vi "Controls Loop.vi"(8 "error in":errorcluster, 10 "Controls[]":refnum<vi>[](array[refnum]), 11 "Material-Scheme in":refnum<class "Material-Scheme.lvclass">) -> (0 "error out":errorcluster)   [LabVIEW 2021, in "TSC Material Theme.lvlib" / "Material-Scheme.lvclass"]
doc: "loop through all the controls on a panel in order to change the appearance\n\n<b>Code Developed By:</b> +\nDaniel Coons +\nTechnology Service Corporation +\nwww.tsc.com/atcs"
uses:
  Material-Scheme.lvclass
  Material-Scheme.lvclass/Material-Scheme.ctl
  <vilib>/Utility/miscctls.llb/LVRowAndColumnTypeDef.ctl
  data member access/Get name.vi
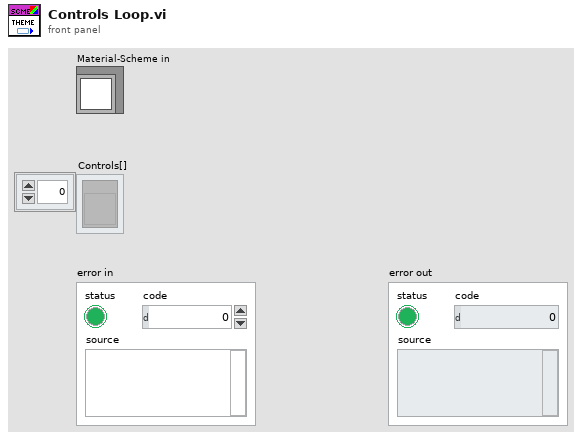
[diagram p1: front panel]
types:
  T1 = typedef "LVRowAndColumnTypeDef.ctl" = cluster{"Row":i32, "Column":i32}
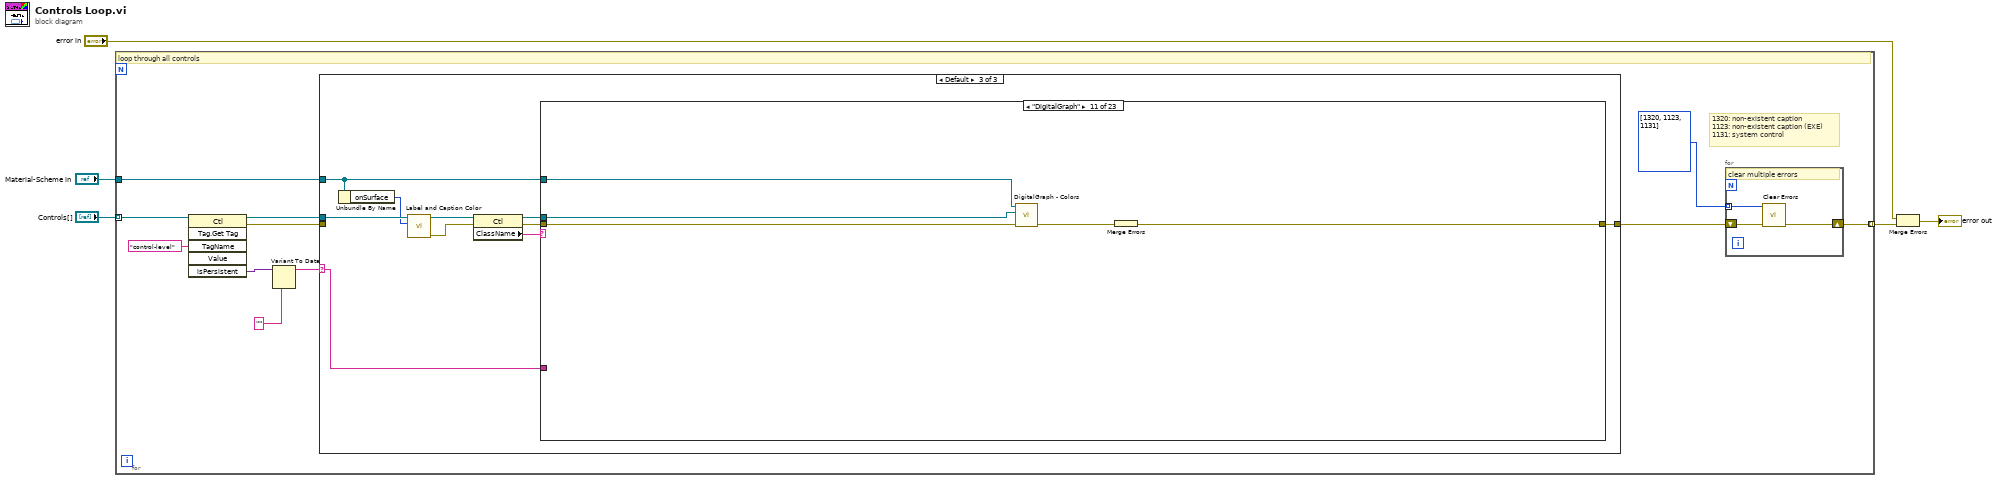
[diagram p0: block diagram]
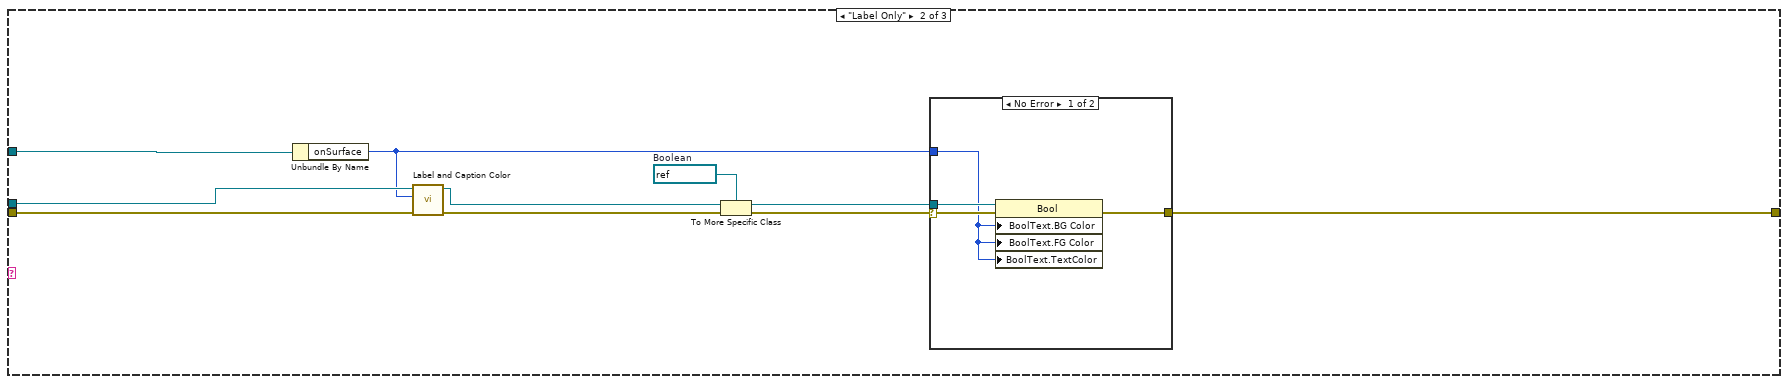
[diagram p3: hidden frame]
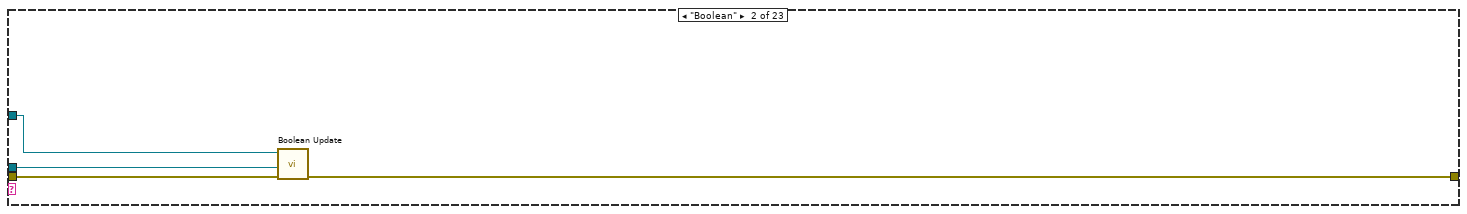
[diagram p6: hidden frame]
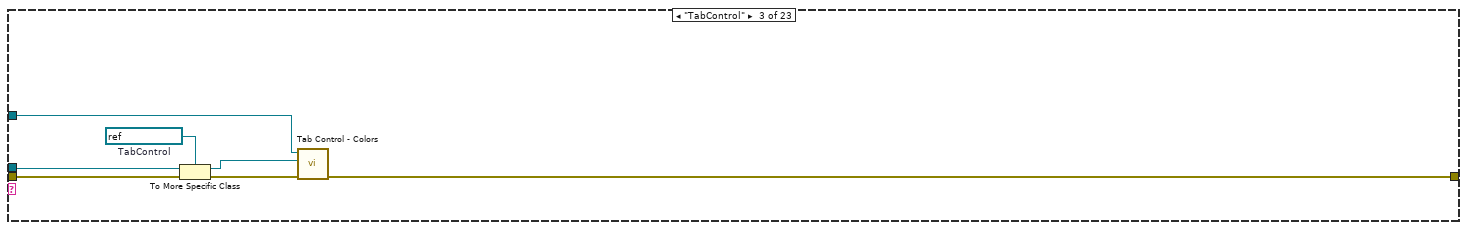
[diagram p7: hidden frame]
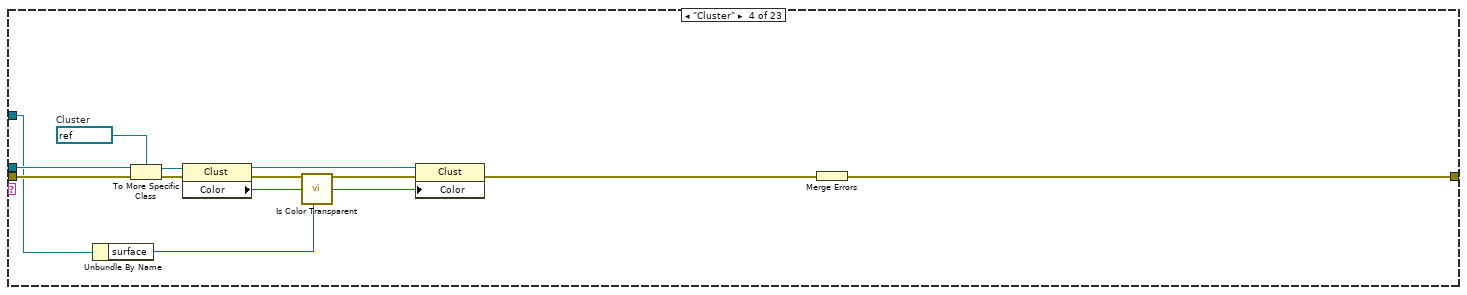
[diagram p8: hidden frame]
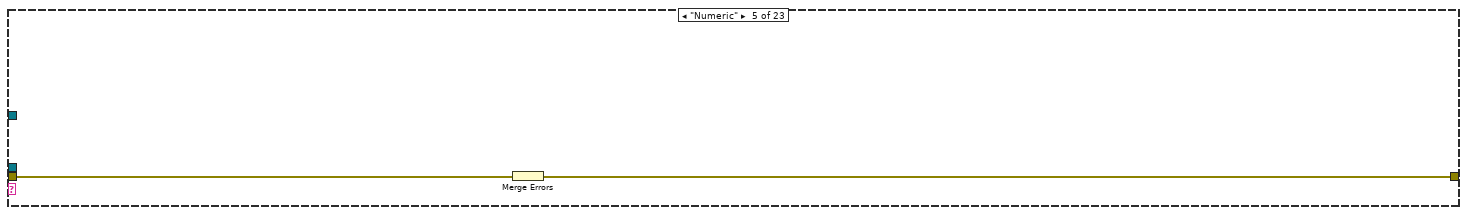
[diagram p9: hidden frame]
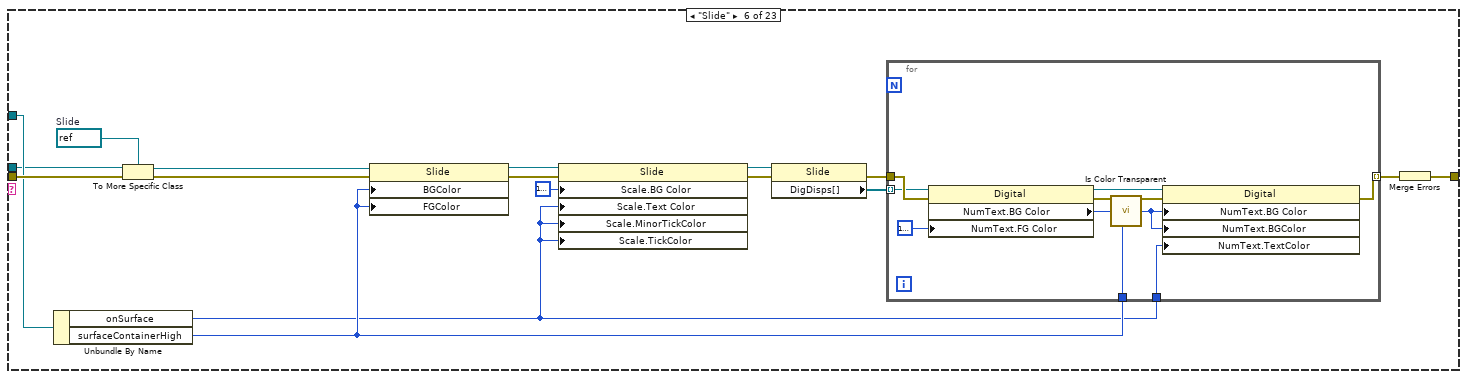
[diagram p10: hidden frame]
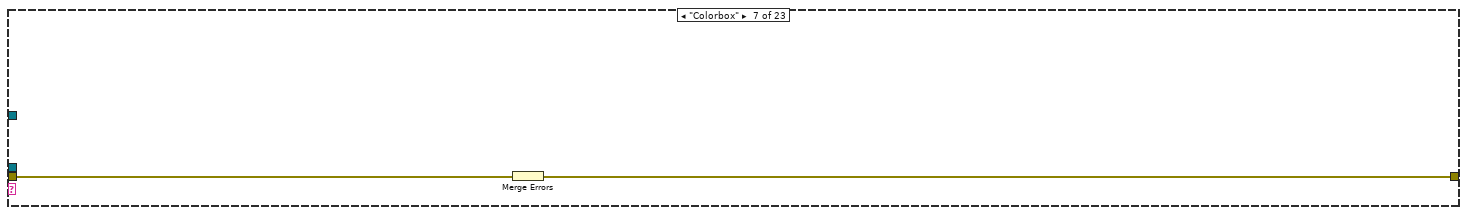
[diagram p11: hidden frame]
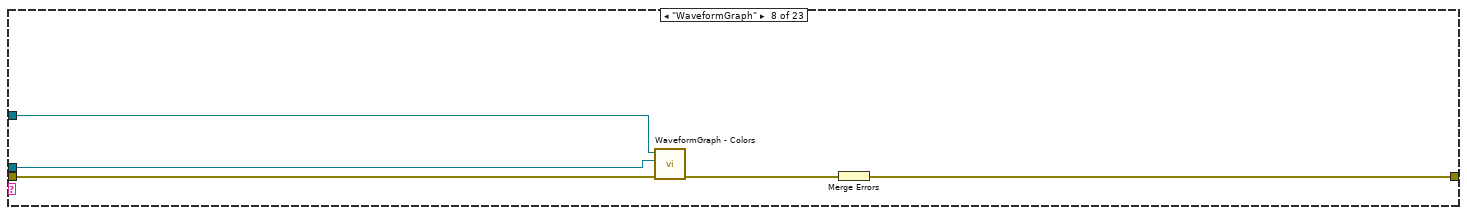
[diagram p12: hidden frame]
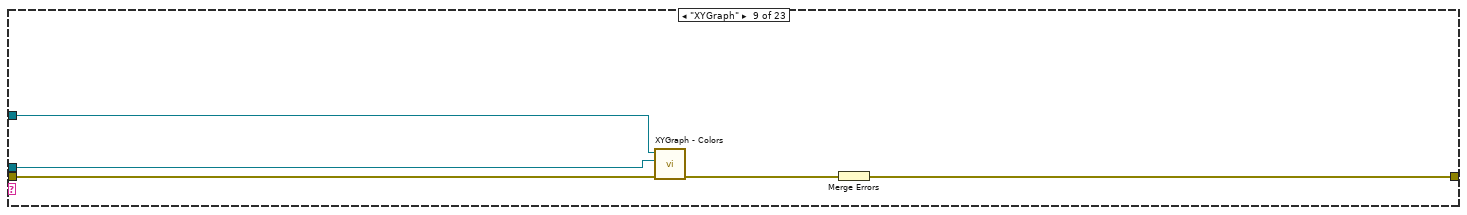
[diagram p13: hidden frame]
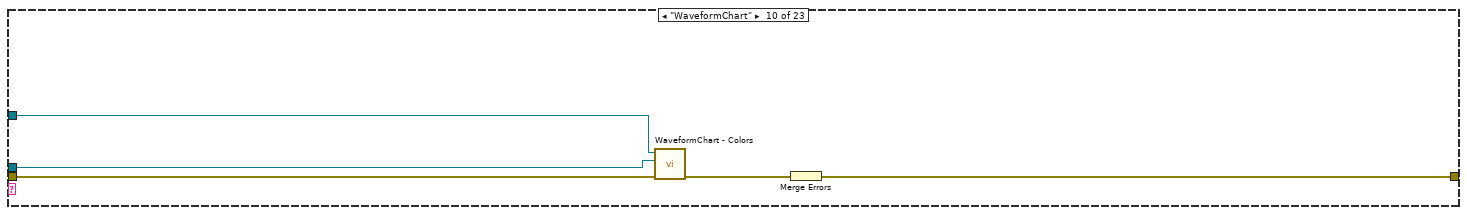
[diagram p14: hidden frame]
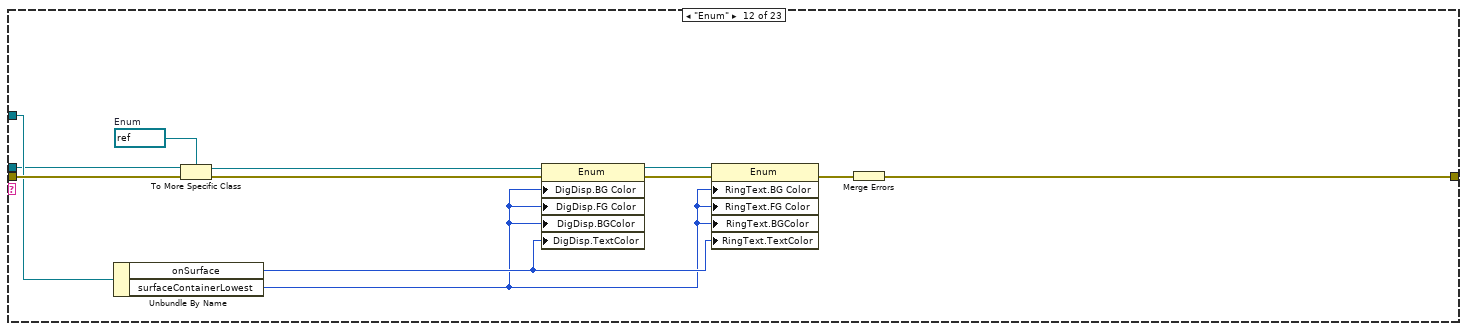
[diagram p15: hidden frame]
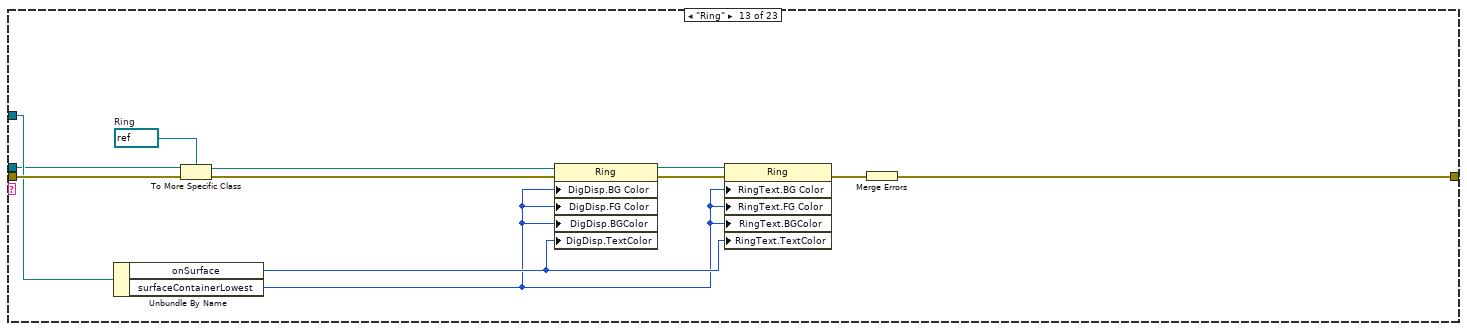
[diagram p16: hidden frame]
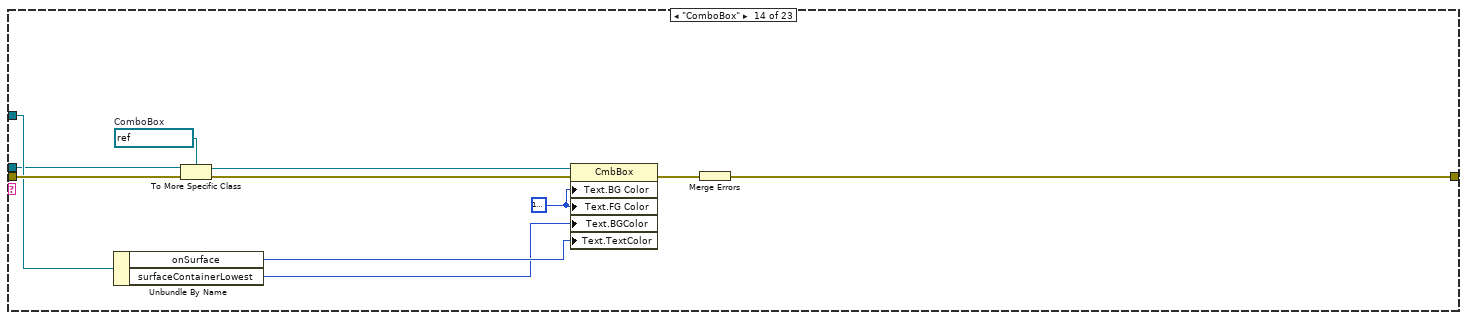
[diagram p17: hidden frame]
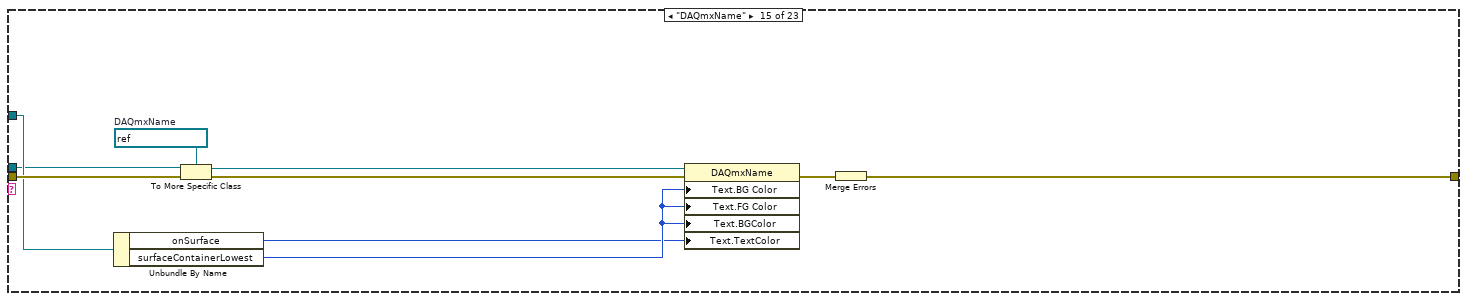
[diagram p18: hidden frame]
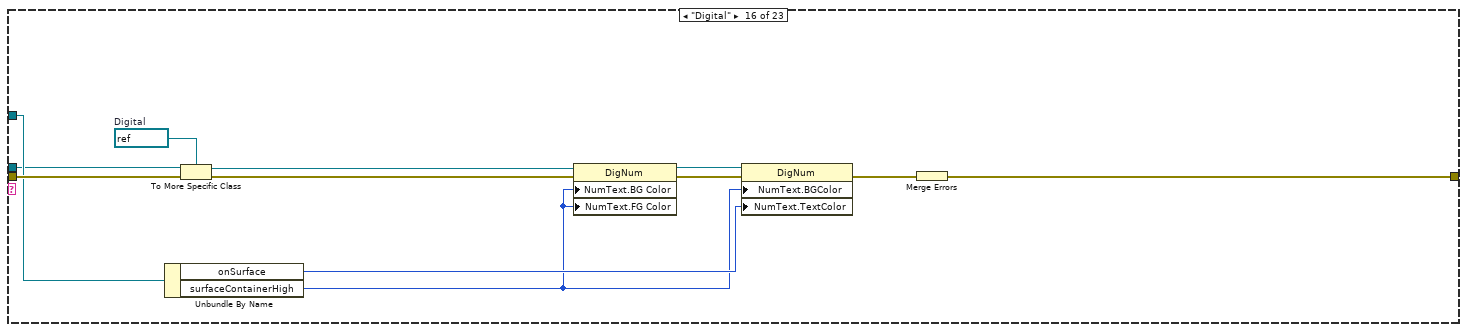
[diagram p19: hidden frame]
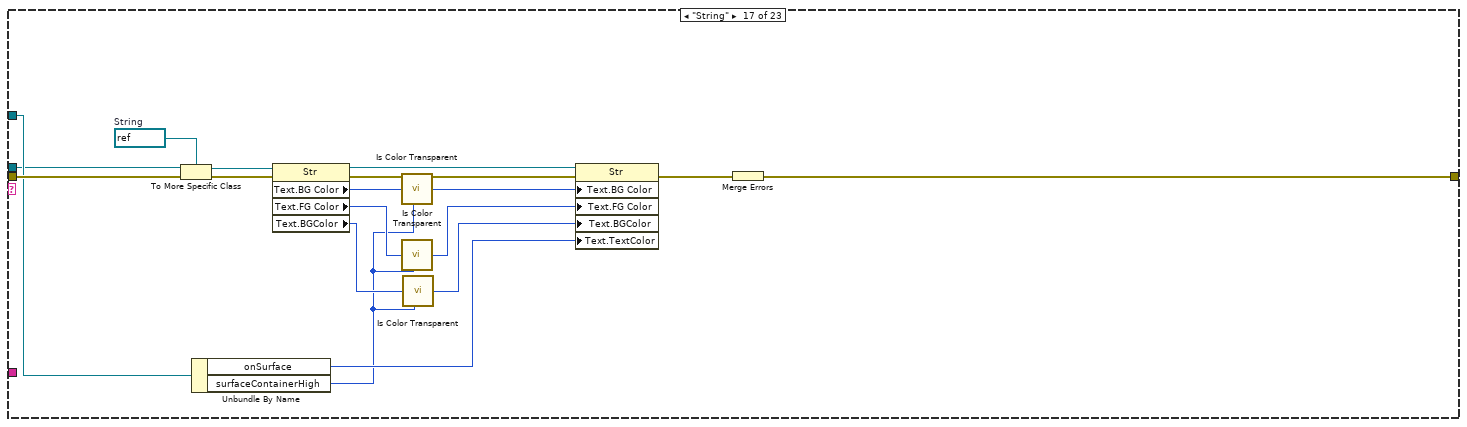
[diagram p20: hidden frame]
diagram:
  n1 = for {
    tunnel: "Controls[]" -> [w13] mode=indexing
    tunnel: "Material-Scheme in" -> [w16]
    tunnel: [w7] -> w3 mode=indexing
    # "1320: non-existent caption\n1123: non-existent caption (EXE)\n1131: system control"
    # "loop through all controls"
    n2 = invoke class="Ctl" method="Tag.Get Tag"(reference=w13, "TagName"="control-level" ("Tag Name")) -> (reference out=w12:refnum<vi>, error out=w8:errorcluster, "isPersistent"=w11:variant)  [unwired: 4 in, 3 out]
    n3 = Variant To Data(type="", Variant=w11) -> (data=w9:string)  [unwired: 1 in, 1 out]
    n4 = case shown="Default" w9 {
      selector: w9 -> [_ _ w37]
      tunnel: w12 -> [_ w20 w36]
      tunnel: w16 -> [_ w26 w33]
      tunnel: [w17 w22 w38] -> w15
      tunnel: w8 -> [w17 w27 _]
      frame "N/A", "no change", "no-change" {
      }
      frame "Label Only" {
        w25 = refnum<vi> refnum  # Boolean
        n5 = Unbundle By Name(w26) -> ("onSurface"=w18:u32)
        n6 = call "Label and Caption Color.vi"("error in"=w27, "Text Color"=w18, "ctrl ref in"=w20) -> ("error out"=w21:errorcluster, "ctrl ref out"=w19:refnum<vi>)  [unwired: 7 in]
        n7 = To More Specific Class(target class=w25, reference=w19, error in=w21) -> (specific class reference=w24:refnum<vi>, error out=w23:errorcluster)
        n8 = case shown="No Error" w23 {
          selector: w23 -> [w30 _]
          tunnel: w24 -> [w31 _]
          tunnel: w18 -> [w29 _]
          tunnel: [w28 _] -> w22
          frame No Error {
            n9 = property class="Bool"(reference=w31, error in=w30, "BoolText.BG Color"=w29, "BoolText.FG Color"=w29, "BoolText.TextColor"=w29) -> (error out=w28:errorcluster)  [unwired: 1 out]
          }
          frame Error {
          }
        }
      }
      frame Default {
        n10 = Unbundle By Name(w33) -> ("onSurface"=w32:u32)
        n11 = call "Label and Caption Color.vi"("Text Color"=w32, "ctrl ref in"=w36) -> ("error out"=w34:errorcluster, "ctrl ref out"=w35:refnum<vi>)  [unwired: 8 in]
        n12 = property class="Ctl"(reference=w35, error in=w34) -> (reference out=w40:refnum<vi>, error out=w39:errorcluster, "ClassName"=w41:string)
        n13 = case shown="\"DigitalGraph\"" w41 {
          tunnel: w40 -> [_ w43 w49 w65 _ w83 _ w99 w104 w109 w114 w125 w137 w148 w158 w170 w187 w196 w206 w217 w239 w266 w286]
          tunnel: w39 -> [w42 w46 w50 w64 w68 w85 w97 w102 w107 w112 w117 w129 w141 w152 w162 w174 w192 w197 w205 w218 w240 w267 w287]
          tunnel: w33 -> [_ w45 w52 w61 _ w84 _ w100 w105 w110 w115 w127 w139 w150 w160 w172 w189 _ w202 w210 w233 w255 w273]
          tunnel: [w42 w44 w53 w62 w67 w71 w96 w101 w106 w111 w116 w128 w140 w151 w161 w173 w191 w194 w203 w212 w222 w257 w275] -> w38
          tunnel: w37 -> [_ _ _ _ _ _ _ _ _ _ _ _ _ _ _ _ _ _ _ w209 w234 w254 w272]
          frame Default {
          }
          frame "Boolean" {
            n14 = call "Boolean Update.vi"("error in (no error)"=w46, "Control in"=w43, "Material-Scheme.lvclass"=w45) -> ("error out"=w44:errorcluster)  [unwired: 8 in]
          }
          frame "TabControl" {
            w51 = refnum<vi> refnum  # TabControl
            n15 = To More Specific Class(target class=w51, reference=w49, error in=w50) -> (specific class reference=w48:refnum<vi>, error out=w47:errorcluster)
            n16 = call "Tab Control - Colors.vi"("error in (no error)"=w47, "ctrl ref in"=w48, "Material-Scheme in"=w52) -> ("error out"=w53:errorcluster)  [unwired: 8 in]
          }
          frame "Cluster" {
            w66 = refnum<vi> refnum  # Cluster
            n17 = Unbundle By Name(w61) -> ("surface"=w55:u32)
            n18 = To More Specific Class(target class=w66, reference=w65, error in=w64) -> (specific class reference=w59:refnum<vi>, error out=w63:errorcluster)
            n19 = property class="Clust"(reference=w59, error in=w63) -> (reference out=w58:refnum<vi>, error out=w60:errorcluster, "Color"=w56:u32)
            n20 = call "Is Color Transparent.vi"("original color"=w56, "desired color"=w55) -> ("updated color"=w57:u32)  [unwired: 3 in]
            n21 = property class="Clust"(reference=w58, error in=w60, "Color"=w57) -> (error out=w54:errorcluster)  [unwired: 1 out]
            n22 = Merge Errors(w54) -> (w62:errorcluster)
          }
          frame "Numeric" {
            n23 = Merge Errors(w68) -> (w67:errorcluster)
          }
          frame "Slide" {
            w82 = refnum<vi> refnum  # Slide
            n24 = Unbundle By Name(w84) -> ("onSurface"=w73:u32, "surfaceContainerHigh"=w74:u32)
            n25 = To More Specific Class(target class=w82, reference=w83, error in=w85) -> (specific class reference=w69:refnum<vi>, error out=w70:errorcluster)
            n26 = property class="Slide"(reference=w69, error in=w70, "BGColor"=w74, "FGColor"=w74) -> (reference out=w80:refnum<vi>, error out=w81:errorcluster)
            n27 = property class="Slide"(reference=w80, error in=w81, "Scale.BG Color"=u32 16777216 ("Scale.Marker Colors:BG Color"), "Scale.Text Color"=w73, "Scale.MinorTickColor"=w73, "Scale.TickColor"=w73) -> (reference out=w77:refnum<vi>, error out=w78:errorcluster)
            n28 = property class="Slide"(reference=w77, error in=w78) -> (error out=w76:errorcluster, "DigDisps[]"=w75:refnum<vi>[])  [unwired: 1 out]
            n29 = for {
              tunnel: w76 -> [w95]
              tunnel: w75 -> [w94] mode=indexing
              tunnel: w74 -> [w90]
              tunnel: w73 -> [w87]
              tunnel: [w86] -> w72 mode=indexing
              n30 = property class="Digital"(reference=w94, error in=w95, "NumText.FG Color"=u32 16777216 ("Numeric Text.Colors:FG Color")) -> (reference out=w92:refnum<vi>, error out=w91:errorcluster, "NumText.BG Color"=w89:u32)
              n31 = call "Is Color Transparent.vi"("original color"=w89, "desired color"=w90) -> ("updated color"=w88:u32)  [unwired: 3 in]
              n32 = property class="Digital"(reference=w92, error in=w91, "NumText.BG Color"=w88, "NumText.BGColor"=w88, "NumText.TextColor"=w87) -> (error out=w86:errorcluster)  [unwired: 1 out]
            }
            n33 = Merge Errors(w72) -> (w71:errorcluster)
          }
          frame "Colorbox" {
            n34 = Merge Errors(w97) -> (w96:errorcluster)
          }
          frame "WaveformGraph" {
            n35 = call "WaveformGraph - Colors.vi"("error in"=w102, "Ctl Refnum"=w99, "Material-Scheme in"=w100) -> ("error out"=w98:errorcluster)  [unwired: 8 in]
            n36 = Merge Errors(w98) -> (w101:errorcluster)
          }
          frame "XYGraph" {
            n37 = call "XYGraph - Colors.vi"("error in"=w107, "Ctl Refnum"=w104, "Material-Scheme in"=w105) -> ("error out"=w103:errorcluster)  [unwired: 8 in]
            n38 = Merge Errors(w103) -> (w106:errorcluster)
          }
          frame "WaveformChart" {
            n39 = call "WaveformChart - Colors.vi"("error in (no error)"=w112, "Ctl Refnum"=w109, "Material-Scheme in"=w110) -> ("error out"=w108:errorcluster)  [unwired: 8 in]
            n40 = Merge Errors(w108) -> (w111:errorcluster)
          }
          frame "DigitalGraph" {
            n41 = call "DigitalGraph - Colors.vi"("error in (no error)"=w117, "Ctl Refnum"=w114, "Material-Scheme in"=w115) -> ("error out"=w113:errorcluster)  [unwired: 8 in]
            n42 = Merge Errors(w113) -> (w116:errorcluster)
          }
          frame "Enum" {
            w123 = refnum<vi> refnum  # Enum
            n43 = Unbundle By Name(w127) -> ("onSurface"=w121:u32, "surfaceContainerLowest"=w119:u32)
            n44 = To More Specific Class(target class=w123, reference=w125, error in=w129) -> (specific class reference=w124:refnum<vi>, error out=w126:errorcluster)
            n45 = property class="Enum"(reference=w124, error in=w126, "DigDisp.BG Color"=w119, "DigDisp.FG Color"=w119, "DigDisp.BGColor"=w119, "DigDisp.TextColor"=w121) -> (reference out=w118:refnum<vi>, error out=w122:errorcluster)
            n46 = property class="Enum"(reference=w118, error in=w122, "RingText.BG Color"=w119, "RingText.FG Color"=w119, "RingText.BGColor"=w119, "RingText.TextColor"=w121) -> (error out=w120:errorcluster)  [unwired: 1 out]
            n47 = Merge Errors(w120) -> (w128:errorcluster)
          }
          frame "Ring" {
            w135 = refnum<vi> refnum  # Ring
            n48 = Unbundle By Name(w139) -> ("onSurface"=w133:u32, "surfaceContainerLowest"=w131:u32)
            n49 = To More Specific Class(target class=w135, reference=w137, error in=w141) -> (specific class reference=w136:refnum<vi>, error out=w138:errorcluster)
            n50 = property class="Ring"(reference=w136, error in=w138, "DigDisp.BG Color"=w131, "DigDisp.FG Color"=w131, "DigDisp.BGColor"=w131, "DigDisp.TextColor"=w133) -> (reference out=w130:refnum<vi>, error out=w134:errorcluster)
            n51 = property class="Ring"(reference=w130, error in=w134, "RingText.BG Color"=w131, "RingText.FG Color"=w131, "RingText.BGColor"=w131, "RingText.TextColor"=w133) -> (error out=w132:errorcluster)  [unwired: 1 out]
            n52 = Merge Errors(w132) -> (w140:errorcluster)
          }
          frame "ComboBox" {
            w142 = u32 16777216 ("Text.Colors:FG Color")
            w146 = refnum<vi> refnum  # ComboBox
            n53 = Unbundle By Name(w150) -> ("onSurface"=w144:u32, "surfaceContainerLowest"=w143:u32)
            n54 = To More Specific Class(target class=w146, reference=w148, error in=w152) -> (specific class reference=w147:refnum<vi>, error out=w149:errorcluster)
            n55 = property class="CmbBox"(reference=w147, error in=w149, "Text.BG Color"=w142, "Text.FG Color"=w142, "Text.BGColor"=w143, "Text.TextColor"=w144) -> (error out=w145:errorcluster)  [unwired: 1 out]
            n56 = Merge Errors(w145) -> (w151:errorcluster)
          }
          frame "DAQmxName" {
            w156 = refnum<vi> refnum  # DAQmxName
            n57 = Unbundle By Name(w160) -> ("onSurface"=w153:u32, "surfaceContainerLowest"=w154:u32)
            n58 = To More Specific Class(target class=w156, reference=w158, error in=w162) -> (specific class reference=w157:refnum<vi>, error out=w159:errorcluster)
            n59 = property class="DAQmxName"(reference=w157, error in=w159, "Text.BG Color"=w154, "Text.FG Color"=w154, "Text.BGColor"=w154, "Text.TextColor"=w153) -> (error out=w155:errorcluster)  [unwired: 1 out]
            n60 = Merge Errors(w155) -> (w161:errorcluster)
          }
          frame "Digital" {
            w168 = refnum<vi> refnum  # Digital
            n61 = Unbundle By Name(w172) -> ("onSurface"=w164:u32, "surfaceContainerHigh"=w163:u32)
            n62 = To More Specific Class(target class=w168, reference=w170, error in=w174) -> (specific class reference=w169:refnum<vi>, error out=w171:errorcluster)
            n63 = property class="DigNum"(reference=w169, error in=w171, "NumText.BG Color"=w163, "NumText.FG Color"=w163) -> (reference out=w165:refnum<vi>, error out=w167:errorcluster)
            n64 = property class="DigNum"(reference=w165, error in=w167, "NumText.BGColor"=w163, "NumText.TextColor"=w164) -> (error out=w166:errorcluster)  [unwired: 1 out]
            n65 = Merge Errors(w166) -> (w173:errorcluster)
          }
          frame "String" {
            w186 = refnum<vi> refnum  # String
            n66 = To More Specific Class(target class=w186, reference=w187, error in=w192) -> (specific class reference=w183:refnum<vi>, error out=w188:errorcluster)
            n67 = Unbundle By Name(w189) -> ("onSurface"=w185:u32, "surfaceContainerHigh"=w178:u32)
            n68 = property class="Str"(reference=w183, error in=w188) -> (reference out=w182:refnum<vi>, error out=w184:errorcluster, "Text.BG Color"=w181:u32, "Text.FG Color"=w180:u32, "Text.BGColor"=w179:u32)
            n69 = call "Is Color Transparent.vi"("original color"=w181, "desired color"=w178) -> ("updated color"=w175:u32)  [unwired: 3 in]
            n70 = call "Is Color Transparent.vi"("original color"=w180, "desired color"=w178) -> ("updated color"=w176:u32)  [unwired: 3 in]
            n71 = call "Is Color Transparent.vi"("original color"=w179, "desired color"=w178) -> ("updated color"=w177:u32)  [unwired: 3 in]
            n72 = property class="Str"(reference=w182, error in=w184, "Text.BG Color"=w175, "Text.FG Color"=w176, "Text.BGColor"=w177, "Text.TextColor"=w185) -> (error out=w190:errorcluster)  [unwired: 1 out]
            n73 = Merge Errors(w190) -> (w191:errorcluster)
          }
          frame "Array" {
            w195 = refnum<vi> refnum  # Array
            n74 = To More Specific Class(target class=w195, reference=w196, error in=w197) -> (error out=w193:errorcluster)  [unwired: 1 out]
            n75 = Merge Errors(w193) -> (w194:errorcluster)
          }
          frame "Path" {
            w207 = refnum<vi> refnum  # Path
            n76 = Unbundle By Name(w202) -> ("surfaceContainerHigh"=w200:u32, "onSurface"=w198:u32)
            n77 = To More Specific Class(target class=w207, reference=w206, error in=w205) -> (specific class reference=w201:refnum<vi>, error out=w204:errorcluster)
            n78 = property class="Path"(reference=w201, error in=w204, "Text.BG Color"=w200, "Text.FG Color"=w200, "Text.FontColor"=w198, "Text.BGColor"=w200, "Text.TextColor"=w198) -> (error out=w199:errorcluster)  [unwired: 1 out]
            n79 = Merge Errors(w199) -> (w203:errorcluster)
          }
          frame "ListBox" {
            w219 = refnum<vi> refnum  # ListBox
            n80 = To More Specific Class(target class=w219, reference=w217, error in=w218) -> (specific class reference=w215:refnum<vi>, error out=w216:errorcluster)
            n81 = call "Color Grabber.vi"("control-level"=w209, "Material-Scheme in"=w210) -> ("colorContainer"=w208:u32)  [unwired: 3 in, 6 out]
            n82 = Unbundle By Name(w210) -> ("surfaceContainerLowest"=w213:u32, "onSurface"=w211:u32)
            n83 = property class="LstBox"(reference=w215, error in=w216, "Active Row"=-2 ("Active Row:Active Row Number"), "CellBG"=w213, "CellFontColor"=w211, "SelColor"=w208) -> (error out=w212:errorcluster)  [unwired: 1 out]
          }
          frame "TreeControl" {
            w236 = -2 ("Active Row:Active Row Number")
            w241 = refnum<vi> refnum  # TreeControl
            n84 = Unbundle By Name(w233) -> ("surfaceContainerLowest"=w235:u32, "onSurface"=w221:u32)
            n85 = To More Specific Class(target class=w241, reference=w239, error in=w240) -> (specific class reference=w237:refnum<vi>, error out=w238:errorcluster)
            n86 = call "Color Grabber.vi"("control-level"=w234, "Material-Scheme in"=w233) -> ("onColor"=w223:u32, "color"=w224:u32, "colorContainer"=w220:u32)  [unwired: 3 in, 4 out]
            n87 = property class="Tree"(reference=w237, error in=w238, "Active Item Row Number"=w236, "ActiveColNum"=w236, "CellBG"=w235, "CellFontColor"=w221, "SelColor"=w220) -> (reference out=w231:refnum<vi>, error out=w232:errorcluster)
            n88 = property class="Tree"(reference=w231, error in=w232, "Active Item Row Number"=-1 ("Active Row:Active Row Number"), "ActiveColNum"=-2 ("Active Row:Active Row Number"), "CellBG"=w224, "CellFontColor"=w223) -> (reference out=w227:refnum<vi>, error out=w228:errorcluster)
            n89 = property class="Tree"(reference=w227, error in=w228, "Active Item Row Number"=-2 ("Active Row:Active Row Number"), "ActiveColNum"=-1 ("Active Row:Active Row Number"), "CellBG"=w224, "CellFontColor"=w223) -> (error out=w222:errorcluster)  [unwired: 1 out]
          }
          frame "MulticolumnListbox" {
            w268 = refnum<vi> refnum  # MulticolumnListbox
            # "check for variations of dark\nand remove horizontal lines"
            # "header"
            n90 = To More Specific Class(target class=w268, reference=w266, error in=w267) -> (specific class reference=w264:refnum<vi>, error out=w265:errorcluster)
            n91 = Unbundle By Name(w255) -> ("surfaceContainerLowest"=w262:u32, "onSurface"=w256:u32)
            n92 = call "Color Grabber.vi"("control-level"=w254, "Material-Scheme in"=w255) -> ("onColor"=w249:u32, "color"=w250:u32, "colorContainer"=w246:u32)  [unwired: 3 in, 4 out]
            n93 = property class="Material-Scheme"(reference=w255) -> ("data member access:name"=w258:string)  [unwired: 1 in, 2 out]
            n94 = property class="MCListbox"(reference=w264, error in=w265, "ActiveCell"=T1 {"Row"=-2, "Column"=-2} ("Active Cell:Active Cell"), "CellBG"=w262, "CellFontColor"=w256) -> (reference out=w260:refnum<vi>, error out=w261:errorcluster)
            n95 = To Lower Case(string=w258) -> (all lower case string=w245:string)
            n96 = property class="MCListbox"(reference=w260, error in=w261, "ActiveCell"=T1 {"Row"=-1, "Column"=-2} ("Active Cell:Active Cell"), "CellBG"=w250, "CellFontColor"=w249, "SelColor"=w246) -> (reference out=w252:refnum<vi>, error out=w253:errorcluster)
            n97 = property class="MCListbox"(reference=w252, error in=w253, "ActiveCell"=T1 {"Row"=-2, "Column"=-1} ("Active Cell:Active Cell"), "CellBG"=w250, "CellFontColor"=w249, "SelColor"=w246) -> (reference out=w247:refnum<vi>, error out=w248:errorcluster)
            n98 = Match Pattern(string=w245, regular expression="dark" ("y")) -> (offset past match=w243:i32)  [unwired: 1 in, 3 out]
            n99 = Less Than 0?(x=w243) -> (x < 0?=w242:bool)
            n100 = property class="MCListbox"(reference=w247, error in=w248, "Horizontal Lines Visible"=w242) -> (error out=w257:errorcluster)  [unwired: 1 out]
          }
          frame "Table" {
            w288 = refnum<vi> refnum  # Table
            n101 = To More Specific Class(target class=w288, reference=w286, error in=w287) -> (specific class reference=w284:refnum<vi>, error out=w285:errorcluster)
            n102 = Unbundle By Name(w273) -> ("surfaceContainerLowest"=w282:u32, "onSurface"=w278:u32)
            n103 = call "Color Grabber.vi"("control-level"=w272, "Material-Scheme in"=w273) -> ("onColor"=w270:u32, "color"=w271:u32, "colorContainer"=w269:u32)  [unwired: 3 in, 4 out]
            n104 = property class="Tbl"(reference=w284, error in=w285, "Active Cell"=T1 {"Row"=-2, "Column"=-2} ("Active Cell:Active Cell"), "Cell BG Color"=w282, "CellFontColor"=w278) -> (reference out=w280:refnum<vi>, error out=w281:errorcluster)
            n105 = property class="Tbl"(reference=w280, error in=w281, "Active Cell"=T1 {"Row"=-1, "Column"=-2} ("Active Cell:Active Cell"), "Cell BG Color"=w271, "CellFontColor"=w270, "Selection Color"=w269) -> (reference out=w276:refnum<vi>, error out=w277:errorcluster)
            n106 = property class="Tbl"(reference=w276, error in=w277, "Active Cell"=T1 {"Row"=-2, "Column"=-1} ("Active Cell:Active Cell"), "Cell BG Color"=w271, "CellFontColor"=w270, "Selection Color"=w269) -> (error out=w275:errorcluster)  [unwired: 1 out]
          }
        }
      }
    }
    n107 = for {
      shift-right: [w290] -> w7
      shift-left: w15 -> [w291]
      tunnel: i32[] [1320, 1123, 1131] -> [w289] mode=indexing
      # "clear multiple errors"
      n108 = call <vilib>:"Clear Errors.vi"("error in (no error)"=w291, "specific error code to clear (0: all)"=w289) -> ("error out"=w290:errorcluster)  [unwired: 4 in, 1 out]
    }
  }
  n109 = Merge Errors("error in", w3) -> (→"error out":errorcluster)
